vi "PSLDAQ_ReadStatus.vi"(0 "Handle In":T1) -> (1 "Status":u32[](array[numeric]), 2 "# Read":i32)   [LabVIEW 2010]
doc: "1. 설명\n a. 통신 연결 상태 및 통신시 발생하는 Event 정보를 획득\n\n2. 기능\n 1. 통신 연결 상태에 대한 정보 획득\n 2. 통신시 상태 변화가 있을 경우 정보 획득 \n \n3. 터미널\n a. 터미널 입력\n ○ Handle In : 장치 핸들 \n\n b. 터미널 출력\n ○ Status : 상태 정보. I32 형태의 배열로 출력됨. 상태 정보는 다음과 같이 분류됨. \n - PS- DAQ 장치와 통신 연결 상태 \n ㆍ1005: 통신 연결 해지됨 \n ㆍ1006: 통신 연결됨 \n - 아날로그 입력 데이터 획득과 관련된 정보 \n ㆍ1001: 데이터 획득(전송) 시작 요청에 대한 응답 받음\n ㆍ1002: 데이터 획득(전송) 중지 요청에 대한 응답 받음\n ㆍ1003: PSL-DAQ 장치의 송신 Queue Overflow\n ㆍ1004: PSLDAQ_DLL.dll의 수신 Queue Overflow \n . 1008: PSLDAQ_DLL.dll에서 데이터 패킷 수신시 패킷 길이 오류 \n\n ○ #Read : 장치로부터 읽은 데이터 샘플 수."
uses:
  PSLDAQ_Dll.dll
panel:
  # "PSLDAQ_ReadStatus\n\n1. 설명\n  a. 통신 연결 상태 및 통신시 발생하는 Event 정보를 획득\n\n2. 기능\n  1. 통신 연결 상태에 대한 정보 획득\n  2. 통신시 상태 변화가 있을 경우 정보 획득 \n     \n3. 터미널\n  a. 터미널 입력\n    ○ Handle In : 장치 핸들 \n\n  b. 터미널 출력\n    ○ Status : 상태 정보. I32 형태의 배열로 출력됨. 상태 정보는 다음과 같이 분류됨. \n        - PS- DAQ 장치와 통신 연결 상태 \n          ㆍ1005: 통신 연결 해지됨 \n          ㆍ1006: 통신 연결됨 \n        -  아날로그 입력 데이터 획득과 관련된 정보 \n          ㆍ1001: 데이터 획득(전송) 시작 요청에 대한 응답 받음\n          ㆍ1002: 데이터 획득(전송) 중지 요청에 대한 응답 받음\n          ㆍ1003: PSL-DAQ 장치의 송신 Queue Overflow\n          ㆍ1004: PSLDAQ_DLL.dll의 수신 Queue Overflow \n           . 1008: PSLDAQ_DLL.dll에서 데이터 패킷 수신시 패킷 길이 오류            \n\n    ○ #Read : 장치로부터 읽은 데이터 샘플 수"
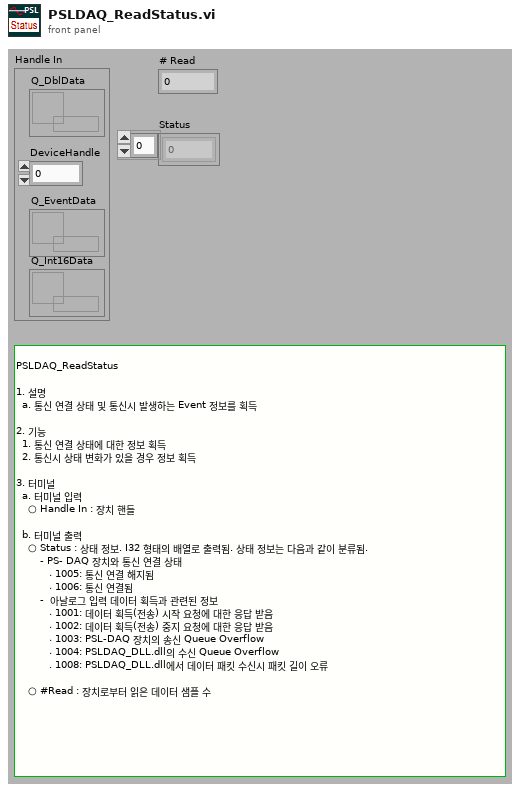
[diagram p1: front panel]
types:
  T1 = cluster{"Q_DblData":refnum<queue>, "DeviceHandle":u32, "Q_EventData":refnum<queue>, "Q_Int16Data":refnum<queue>}
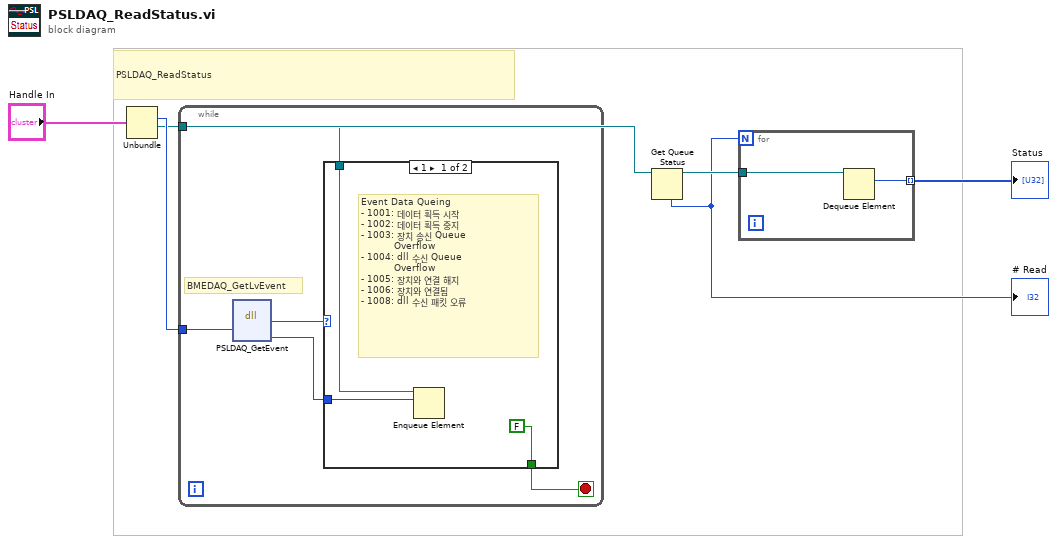
[diagram p0: block diagram]
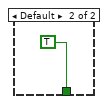
[diagram p2: hidden frame]
diagram:
  # "PSLDAQ_ReadStatus"
  n1 = Unbundle("Handle In") -> ("DeviceHandle"=w3:u32, "Q_EventData"=w2:refnum<queue>)  [unwired: 2 out]
  n2 = while {
    tunnel: w3 -> [w9]
    tunnel: w2 -> [w8]
    stop <- w7 stop-if-true
    # "BMEDAQ_GetLvEvent"
    n3 = dll-call lib="D:/PSL-DAQ LabVIEW Library/PSLDAQ_Dll.dll" fn="PSLDAQ_GetEvent"("DeviceHandle"=w9) -> ("return type"=w11:u8, "EventData"=w10:i32)  [unwired: 5 in, 2 out]
    n4 = case shown="1" w11 {
      tunnel: w10 -> [w14 _]
      tunnel: w8 -> [w13 _]
      tunnel: [FALSE TRUE] -> w7
      frame 1 {
        # "Event Data Queing \n- 1001: 데이터 획득 시작\n- 1002: 데이터 획득 중지\n- 1003: 장치 송신 Queue \n           Overflow\n- 1004: dll 수신 Queue\n           Overflow\n- 1005: 장치와 연결 해지\n- 1006: 장치와 연결됨 \n- 1008: dll 수신 패킷 오류"
        n5 = Enqueue Element(queue=w13, element=w14) -> ()  [unwired: 2 in, 3 out]
      }
      frame Default {
      }
    }
  }
  n6 = Get Queue Status(queue=w2) -> (queue out=w6:refnum<queue>, # elements in queue=w5:i32)  [unwired: 2 in, 6 out]
  "# Read" <- w5
  n7 = for {
    N: w5 -> [_]
    tunnel: w6 -> [w17]
    tunnel: [w16] -> w4 mode=indexing
    n8 = Dequeue Element(queue=w17) -> (element=w16:u32)  [unwired: 2 in, 3 out]
  }
  "Status" <- w4
